vi "rtRPM.vi"(9 "Tach 2 Period (100 us)":dbl, 10 "Tach 1 Period (100 us)":dbl) -> (1 "Avg RPM":dbl, 2 "RPM 2":dbl, 3 "RPM 1":dbl)   [LabVIEW 2019]
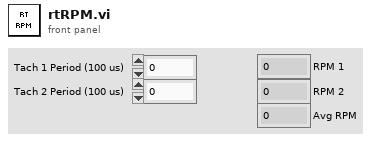
[diagram p1: front panel]
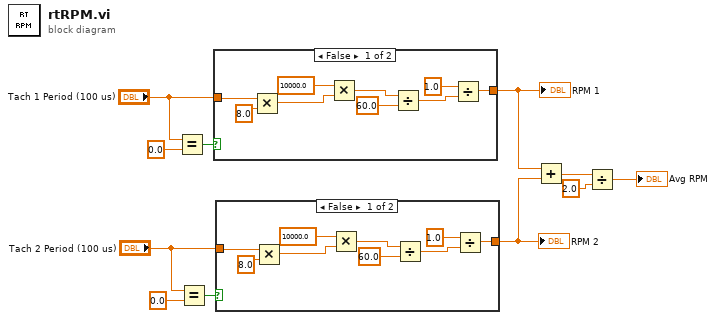
[diagram p0: block diagram]
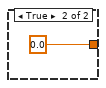
[diagram p2: hidden frame]
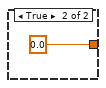
[diagram p3: hidden frame]
diagram:
  n1 = Equal?(x="Tach 1 Period (100 us)", y=0.0) -> (x = y?=w11:bool)
  n2 = Equal?(x="Tach 2 Period (100 us)", y=0.0) -> (x = y?=w8:bool)
  n3 = case shown="False" w11 {
    tunnel: "Tach 1 Period (100 us)" -> [w15 _]
    tunnel: [w13 0.0] -> w4
    frame False {
      n4 = Multiply(x=w15, y=8.0) -> (x*y=w19:dbl)
      n5 = Multiply(x=10000.0, y=w19) -> (x*y=w20:dbl)
      n6 = Divide(x=w20, y=60.0) -> (x/y=w12:dbl)
      n7 = Divide(x=1.0, y=w12) -> (x/y=w13:dbl)
    }
    frame True {
    }
  }
  "RPM 1" <- w4
  n8 = case shown="False" w8 {
    tunnel: "Tach 2 Period (100 us)" -> [w25 _]
    tunnel: [w23 0.0] -> w5
    frame False {
      n9 = Multiply(x=w25, y=8.0) -> (x*y=w29:dbl)
      n10 = Multiply(x=10000.0, y=w29) -> (x*y=w30:dbl)
      n11 = Divide(x=w30, y=60.0) -> (x/y=w22:dbl)
      n12 = Divide(x=1.0, y=w22) -> (x/y=w23:dbl)
    }
    frame True {
    }
  }
  "RPM 2" <- w5
  n13 = Add(x=w4, y=w5) -> (x+y=w2:dbl)
  n14 = Divide(x=w2, y=2.0) -> (x/y=→"Avg RPM":dbl)
